vi "Turn all Colors off.vi"(8 "error in (no error)":errorcluster, 11 "GameLogic in":refnum<class "GameLogic.lvclass">) -> (0 "error out":errorcluster, 3 "GameLogic out":refnum<class "GameLogic.lvclass">)   [LabVIEW 2019, in "GameLogic.lvlib" / "GameLogic.lvclass"]
uses:
  GameLogic.lvclass
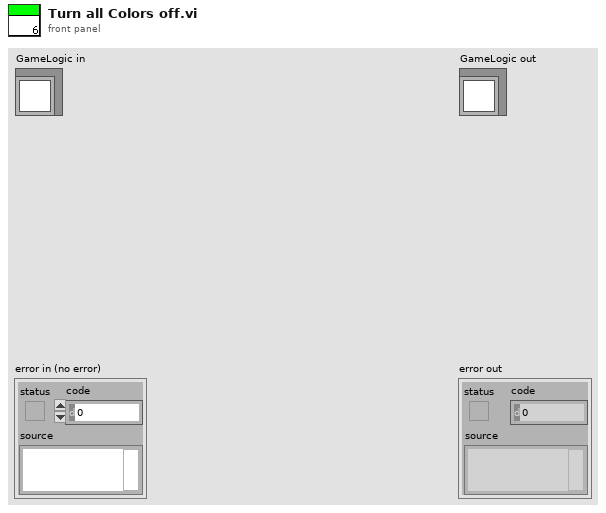
[diagram p1: front panel]
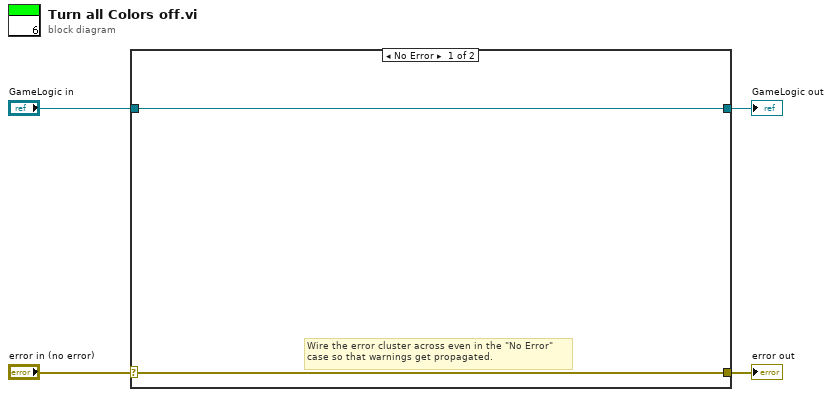
[diagram p0: block diagram]
diagram:
  n1 = case shown="No Error" "error in (no error)" {
    selector: "error in (no error)" -> [w5 w8]
    tunnel: [w5 w8] -> w3
    tunnel: [w6 w7] -> w1
    tunnel: "GameLogic in" -> [w6 w7]
    frame No Error {
      # "Wire the error cluster across even in the \"No Error\"\ncase so that warnings get propagated."
    }
    frame Error {
    }
  }
  "error out" <- w3
  "GameLogic out" <- w1
